vi "Handle UNREGISTERED.vi"(8 "error in (no error)":errorcluster, 9 "WAMP Message":T16 {"Message Codes" items=["HELLO"=1, "WELCOME"=2, "ABORT"=3, "GOODBYE"=6, "ERROR"=8, "PUBLISH"=16, "PUBLISHED"=17, "SUBSCRIBE"=32, "SUBSCRIBED"=33, "UNSUBSCRIBE"=34, "UNSUBSCRIBED"=35, "EVENT"=36, "CALL"=48, "RESULT"=59, "REGISTER"=64, "REGISTERED"=65, "UNREGISTER"=66, "UNREGISTERED"=67, "INVOCATION"=68, "YIELD"=70]}, 10 "Message loop data (in)":T1, 11 "reference":refnum<class "WAMP Client.lvclass">) -> (0 "error out":errorcluster, 2 "Message Loop Data (Out)":T1, 3 "reference out":refnum<class "WAMP Client.lvclass">)   [LabVIEW 2020, in "wamplv.lvlib" / "WAMP Client.lvclass"]
uses:
  WAMP Client.lvclass
  TypeDef/WAMP Received Message.ctl
  TypeDef/WAMP Message Codes.ctl
  TypeDef/Message Loop Shift Reg Data.ctl
  TypeDef/REGISTER Request Data.ctl
  API/TypeDefs/INVOCATION payload.ctl
  TypeDef/Success or error.ctl
  API/TypeDefs/Combined error.ctl
  API/TypeDefs/WAMP error.ctl
  TypeDef/Publish Requests Map.ctl
  TypeDef/PUBLISH Request Data.ctl
  TypeDef/PUBLISH result.ctl
  TypeDef/Endpoint Data.ctl
  TypeDef/CALL Request Map.ctl
  TypeDef/CALL Request Data.ctl
  API/TypeDefs/RESULT payload.ctl
  TypeDef/SUBSCRIBE Requests Map.ctl
  TypeDef/SUBSCRIBE Request Data.ctl
  TypeDef/Subscribe Result.ctl
  TypeDef/EVENT payload.ctl
  TypeDef/Subscriptions Map.ctl
  TypeDef/Subscription Details.ctl
  TypeDef/Unsubscribe Requests Map.ctl
  TypeDef/UNSUBSCRIBE Request Data.ctl
  TypeDef/UNSUBSCRIBE Result.ctl
  TypeDef/Unregister requests map.ctl
  TypeDef/Unregister request.ctl
  WAMP Client.lvclass/WAMP Client.ctl
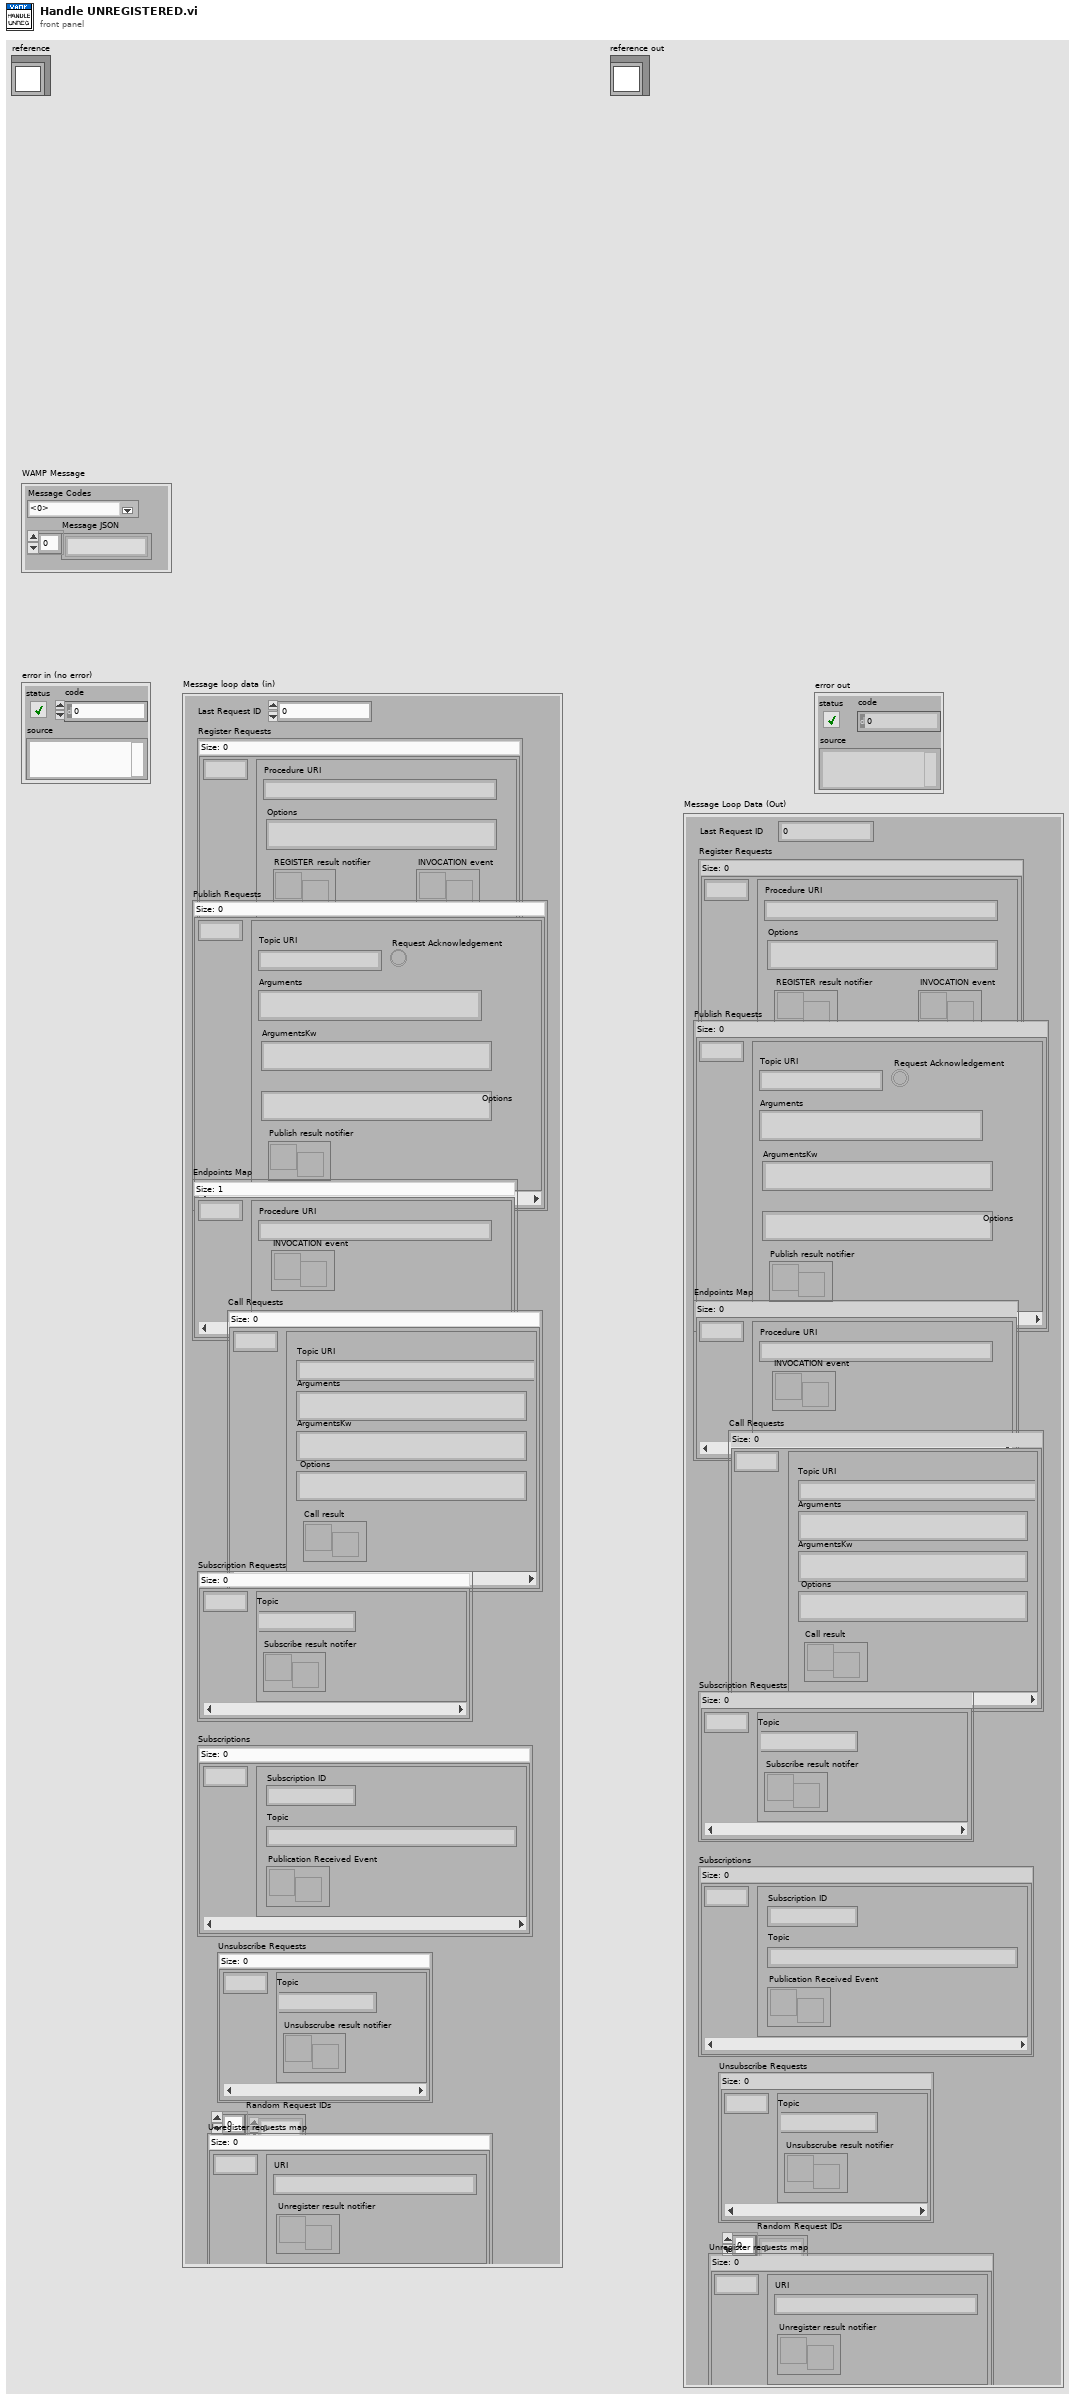
[diagram p1: front panel]
types:
  T1 = typedef "wamplv.lvlib/WAMP Client.lvclass/Message Loop Shift Reg Data.ctl" = cluster{"Last Request ID":u64, "Register Requests":map{u64, T2}, "Publish Requests":T3, "Endpoints Map":map{u64, T5}, "Call Requests":T6, "Subscription Requests":T8, "Subscriptions":T10, "Unsubscribe Requests":T12, "Random Request IDs":u64[], "Unregister requests map":T14}
  T2 = typedef "wamplv.lvlib/WAMP Client.lvclass/REGISTER Request Data.ctl" = cluster{"Procedure URI":string, "Options":string, "INVOCATION event":refnum<user-event>, "REGISTER result notifier":refnum<notifier>}
  T3 = typedef "wamplv.lvlib/WAMP Client.lvclass/Publish Requests Map.ctl" = map{u64, T4}
  T4 = typedef "wamplv.lvlib/WAMP Client.lvclass/PUBLISH Request Data.ctl" = cluster{"Topic URI":string, "Arguments":string, "ArgumentsKw":string, "Request Acknowledgement":bool, "Options":string, "Publish result notifier":refnum<notifier>}
  T5 = typedef "wamplv.lvlib/WAMP Client.lvclass/Endpoint Data.ctl" = cluster{"Procedure URI":string, "INVOCATION event":refnum<user-event>}
  T6 = typedef "wamplv.lvlib/WAMP Client.lvclass/CALL Request Map.ctl" = map{u64, T7}
  T7 = typedef "wamplv.lvlib/WAMP Client.lvclass/CALL Request Data.ctl" = cluster{"Topic URI":string, "Arguments":string, "ArgumentsKw":string, "Options":string, "Call result":refnum<notifier>}
  T8 = typedef "wamplv.lvlib/WAMP Client.lvclass/SUBSCRIBE Requests Map.ctl" = map{u64, T9}
  T9 = typedef "wamplv.lvlib/WAMP Client.lvclass/SUBSCRIBE Request Data.ctl" = cluster{"Topic":string, "Subscribe result notifer":refnum<notifier>}
  T10 = typedef "wamplv.lvlib/WAMP Client.lvclass/Subscriptions Map.ctl" = map{u64, T11}
  T11 = typedef "wamplv.lvlib/WAMP Client.lvclass/Subscription Details.ctl" = cluster{"Subscription ID":u64, "Topic":string, "Publication Received Event":refnum<user-event>}
  T12 = typedef "wamplv.lvlib/WAMP Client.lvclass/Unsubscribe Requests Map.ctl" = map{u64, T13}
  T13 = typedef "wamplv.lvlib/WAMP Client.lvclass/UNSUBSCRIBE Request Data.ctl" = cluster{"Topic":string, "Unsubscrube result notifier":refnum<notifier>}
  T14 = typedef "wamplv.lvlib/WAMP Client.lvclass/Unregister requests map.ctl" = map{u64, T15}
  T15 = typedef "wamplv.lvlib/WAMP Client.lvclass/Unregister request.ctl" = cluster{"URI":string, "Unregister result notifier":refnum<notifier>}
  T16 = typedef "wamplv.lvlib/WAMP Client.lvclass/WAMP Received Message.ctl" = cluster{"Message JSON":string[], "Message Codes":T17}
  T17 = typedef "wamplv.lvlib/WAMP Client.lvclass/WAMP Message Codes.ctl" = u16
  T18 = typedef "wamplv.lvlib/WAMP Client.lvclass/Success or error.ctl" = cluster{"Success?":bool, "URI":string, "Combined Error":T19}
  T19 = typedef "wamplv.lvlib/WAMP Client.lvclass/Combined error.ctl" = cluster{"Error?":bool, "WAMP Error":T20, "Error":errorcluster}
  T20 = typedef "wamplv.lvlib/WAMP Client.lvclass/WAMP error.ctl" = cluster{"Details":string, "ArgumentKw Payload":string, "Error?":bool, "Error URI":string, "Arguments Payload":string}
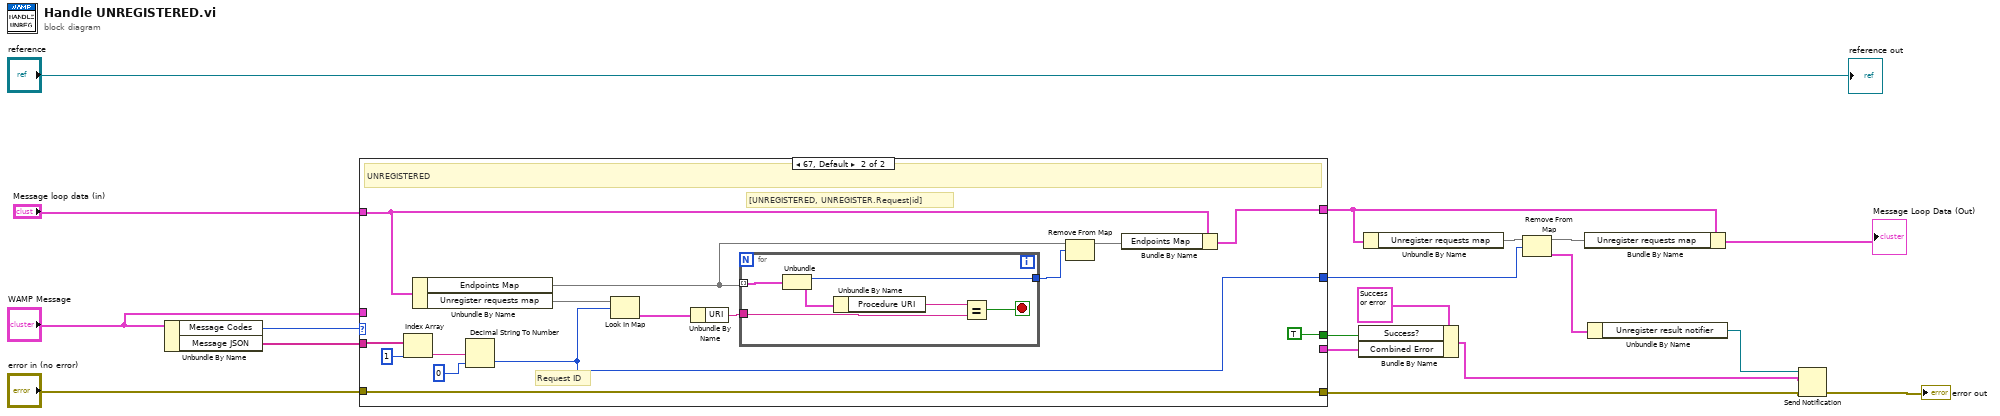
[diagram p0: block diagram]
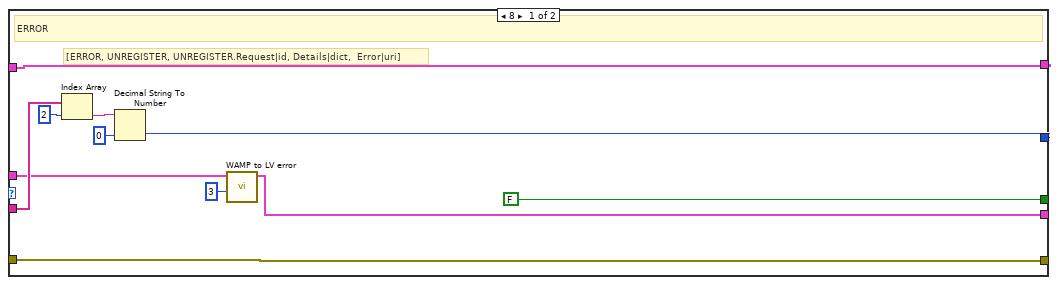
[diagram p2: hidden frame]
diagram:
  n1 = Unbundle By Name("WAMP Message") -> ("Message Codes"=w15:T17, "Message JSON"=w14:string[])
  n2 = case shown="67, Default" w15 {
    tunnel: w14 -> [w28 w44]
    tunnel: [w26 w31] -> w13
    tunnel: "error in (no error)" -> [w27 w43]
    tunnel: [w27 w43] -> w4
    tunnel: [w20 _] -> w18
    tunnel: [FALSE ("Success?") TRUE ("Success?")] -> w17
    tunnel: "Message loop data (in)" -> [w25 w39]
    tunnel: [w25 w38] -> w7
    tunnel: "WAMP Message" -> [w22 _]
    frame 8 {
      # "[ERROR, UNREGISTER, UNREGISTER.Request|id, Details|dict,  Error|uri]"
      # "ERROR"
      n3 = Index Array(array=w28, index=2) -> (element=w29:string)
      n4 = Decimal String To Number(string=w29, default (0L)=u64 0 ("default (0 I32)")) -> (number=w26:u64)  [unwired: 1 in, 1 out]
      n5 = call "WAMP to LV error.vi"("Details Index"=u32 3, "WAMP Message"=w22) -> ("Combined Error"=w20:T19)  [unwired: 7 in, 2 out]
    }
    frame 67, Default {
      # "[UNREGISTERED, UNREGISTER.Request|id]"
      # "Request ID"
      # "UNREGISTERED"
      n6 = Index Array(array=w44, index=1) -> (element=w41:string)
      n7 = Unbundle By Name(w39) -> ("Endpoints Map"=w34:map{u64, T5}, "Unregister requests map"=w35:T14)
      n8 = Decimal String To Number(string=w41, default (0L)=u64 0) -> (number=w31:u64)  [unwired: 1 in, 1 out]
      n9 = Look In Map(map=w35, key=w31) -> (value=w36:T15)  [unwired: 1 in, 1 out]
      n10 = Unbundle By Name(w36) -> ("URI"=w37:string)
      n11 = for {
        tunnel: [w49] -> w32
        tunnel: w34 -> [w47] mode=indexing
        tunnel: w37 -> [w46]
        stop <- w50 stop-if-true
        n12 = Unbundle(w47) -> ("key"=w49:u64, "Endpoint Data"=w51:T5)
        n13 = Unbundle By Name(w51) -> ("Procedure URI"=w48:string)
        n14 = Equal?(x=w48, y=w46) -> (x = y?=w50:bool)
      }
      n15 = Remove From Map(10:w32, 11:w34) -> (3:w33:map{u64, T5})  [unwired: 2 out]
      n16 = Bundle By Name(cluster=w39, "Endpoints Map"=w33) -> (w38:T1)
    }
  }
  n17 = Bundle By Name(cluster=T18 {"Success?"=FALSE, "URI"="", "Combined Error"={"Error?"=FALSE, "WAMP Error"={"Details"="{}", "ArgumentKw Payload"="{}", "Error?"=FALSE, "Error URI"="", "Arguments Payload"=""}, "Error"={"status"=FALSE, "code"=0, "source"=""}}} ("Sucess or error"), "Success?"=w17, "Combined Error"=w18) -> (w2:T18)
  n18 = Unbundle By Name(w7) -> ("Unregister requests map"=w9:T14)
  n19 = Remove From Map(10:w13, 11:w9) -> (1:w12:T15, 3:w10:T14)  [unwired: 1 out]
  n20 = Bundle By Name(cluster=w7, "Unregister requests map"=w10) -> (→"Message Loop Data (Out)":T1)
  n21 = Unbundle By Name(w12) -> ("Unregister result notifier"=w1:refnum<notifier>)
  n22 = Send Notification(notification=w2, notifier=w1, error in (no error)=w4) -> (error out=→"error out":errorcluster)  [unwired: 1 out]
  "reference out" <- "reference"
